vi "Video File Frame Read.vi"(8 "error in (no error)":errorcluster, 10 "Image Dst":T1, 11 "Video Processor in":refnum<class "Video Cam Processor.lvclass">) -> (0 "error out":errorcluster, 2 "Video Frame out":refnum<class "Video Frame.lvclass">, 3 "Video Processor out":refnum<class "Video Cam Processor.lvclass">, 4 "Playback Finished?":bool, 6 "Looped?":bool)   [LabVIEW 2018, in "Video Cam Processor.lvclass"]
uses:
  Video Cam Processor.lvclass
  <vilib>/vision/Image Controls.llb/IMAQ Image.ctl
  Video Frame/Video Frame.lvclass
  Realsense Cam Video File Wrapper/Realsense Cam File Wrapper.lvclass
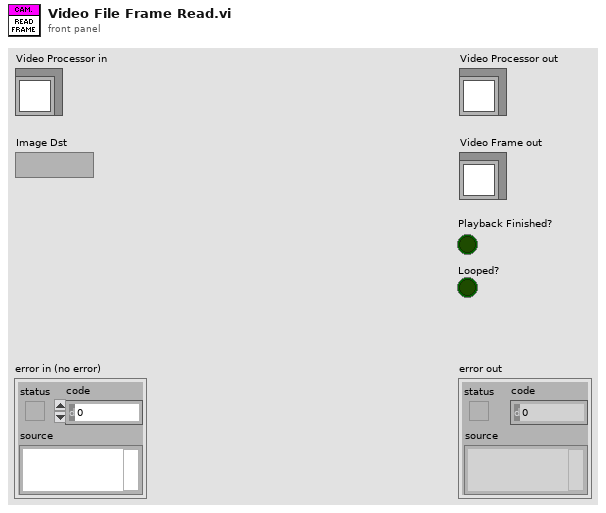
[diagram p1: front panel]
types:
  T1 = typedef "IMAQ Image.ctl" = refnum<image>
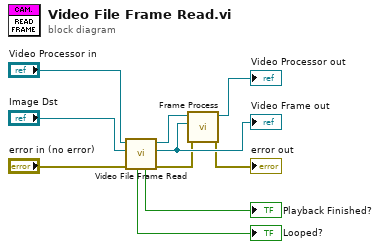
[diagram p0: block diagram]
diagram:
  n1 = call-parent "Video File Frame Read.vi"("error in (no error)"="error in (no error)", "Image Dst"="Image Dst", "Realsense Cam File Wrapper in"="Video Processor in") -> ("error out"=w4:errorcluster, "Video Frame out"=w6:refnum<class "Video Frame.lvclass">, "Realsense Cam File Wrapper out"=w7:refnum<class "Video Cam Processor.lvclass">, "Playback Finished?"=→"Playback Finished?":bool, "Looped?"=→"Looped?":bool)  [unwired: 4 in]
  "Video Frame out" <- w6
  n2 = call-dynamic "Frame Process.vi"("error in (no error)"=w4, "Video Frame In"=w6, "Video Processor in"=w7) -> ("error out"=→"error out":errorcluster, "Video Processor out"=→"Video Processor out":refnum<class "Video Cam Processor.lvclass">)  [unwired: 7 in]
